vi "Check ABORT.vi"(8 "error in":errorcluster) -> (0 "error out":errorcluster, 3 "ABORT?":bool)   [LabVIEW 2020, in "TALOS.lvlib"]
doc: "Use this VI to check the status of the ABORT SV. It is optimised respect to just opening the SV on the network."
uses:
  TALOS.lvlib
  Classes/Circus Shared Variables/Circus Shared Variables.lvclass/Circus Shared Variables.ctl
  Ancestor/Ancestor/Ancestor.lvclass/Ancestor.ctl
  Generate Error.vi
  FGV/Error Memory/Get Error Description.vi
  Get PC name.vi
  Ancestor/Ancestor/Read ID.vi
  Get Class Name.vi
  <vilib>/Utility/error.llb/Clear Errors.vi
  FGV/Error Memory/Error Memory Core.vi
  <vilib>/AdvancedString/Delimited String to 1D String Array.vi
  Circus Root Path.vi
  FGV/Error Memory/Error Crt Lvl checker.vi
  FGV/Error Memory/Error Memory Core.vi/40c8088d-b597-4017-91af-faa98e00292e.vi
  FGV/Error Memory/Error Memory Core.vi/d4a3ab98-063c-4e44-b43d-fbdcfe6c2be2.vi
  Global Constants.vi
  Global Memory.vi
  <vilib>/Utility/LVClass/Get LV Class Name.vi
  Is in Packed Library.vi
  TALOS Root path.vi
  Read CSV worksheet.vi
  <vilib>/Utility/error.llb/General Error Handler.vi
  Error Log.vi
  Ancestor/Ancestor/Ancestor.lvclass
  <vilib>/Comparison/Equal/Equal Functor/Equal Functor.lvclass
  Classes/Circus Shared Variables/Circus Shared Variables.lvclass
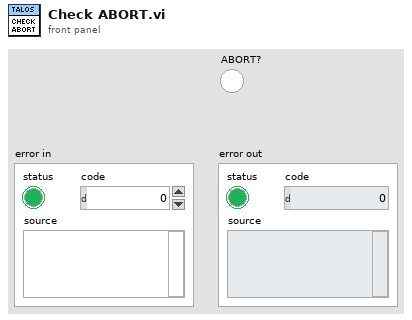
[diagram p1: front panel]
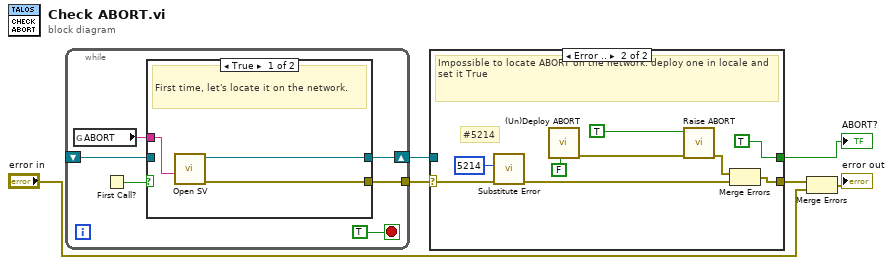
[diagram p0: block diagram]
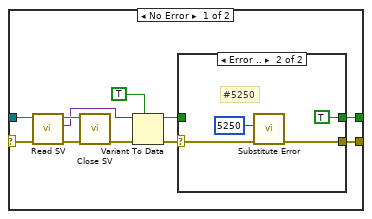
[diagram p2: hidden frame]
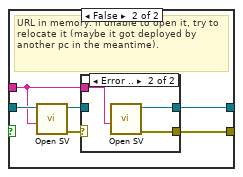
[diagram p4: hidden frame]
diagram:
  n1 = while {
    tunnel: [w12] -> w6
    shift-right: [w11] -> w5
    shift-left: _ -> [w8]
    stop <- TRUE stop-if-true
    n2 = global read "Global Constants.vi" "ABORT"() -> (w7:string)
    n3 = First Call?() -> (First Call?: T/F=w10:bool)
    n4 = case shown="True" w10 {
      tunnel: [w15 w17] -> w12
      tunnel: [w14 w18] -> w11
      tunnel: w8 -> [_ w21]
      tunnel: w7 -> [w13 w16]
      frame True {
        # "First time, let's locate it on the network."
        n5 = call "Open SV.vi"("SV Name"=w13) -> ("error out"=w15:errorcluster, "AEgIS Shared Variables out"=w14:refnum<class "Circus Shared Variables.lvclass">)  [unwired: 9 in]
      }
      frame False {
        # "URL in memory: if unable to open it, try to relocate it (maybe it got deployed by another pc in the meantime)."
        n6 = call "Open SV.vi"("SV Name"=w16, "AEgIS Shared Variables in"=w21) -> ("error out"=w20:errorcluster, "AEgIS Shared Variables out"=w19:refnum<class "Circus Shared Variables.lvclass">)  [unwired: 8 in]
        n7 = case shown="Error .." w20 {
          selector: w20 -> [w22 _]
          tunnel: w19 -> [w23 _]
          tunnel: [w23 w26] -> w18
          tunnel: [w22 w25] -> w17
          tunnel: w16 -> [_ w24]
          frame No Error {
          }
          frame Error {
            n8 = call "Open SV.vi"("SV Name"=w24) -> ("error out"=w25:errorcluster, "AEgIS Shared Variables out"=w26:refnum<class "Circus Shared Variables.lvclass">)  [unwired: 9 in]
          }
        }
      }
    }
  }
  n9 = case shown="Error .." w6 {
    selector: w6 -> [w37 w52]
    tunnel: w5 -> [w34 _]
    tunnel: [w28 TRUE] -> w4
    tunnel: [w27 w45] -> w3
    frame No Error {
      n10 = call "Read SV.vi"("error in (no error)"=w37, "AEgIS Shared Variables in"=w34) -> ("error out"=w36:errorcluster, "Variant"=w32:variant, "AEgIS Shared Variables out"=w35:refnum<class "Circus Shared Variables.lvclass">)  [unwired: 7 in]
      n11 = call "Close SV.vi"("error in (no error)"=w36, "AEgIS Shared Variables in"=w35) -> ("error out"=w33:errorcluster)  [unwired: 7 in, 2 out]
      n12 = Variant To Data(error in=w33, type=TRUE, Variant=w32) -> (data=w29:bool, error out=w30:errorcluster)
      n13 = case shown="Error .." w30 {
        selector: w30 -> [w38 w41]
        tunnel: w29 -> [w39 _]
        tunnel: [w39 TRUE] -> w28
        tunnel: [w38 w40] -> w27
        frame No Error {
        }
        frame Error {
          # "#5250"
          n14 = call "Substitute Error.vi"("error in (no error)"=w41, "Error Code"=5250) -> ("error out"=w40:errorcluster)  [unwired: 9 in]
        }
      }
    }
    frame Error {
      # "#5214"
      # "Impossible to locate ABORT on the network: deploy one in locale and set it True"
      n15 = call "Substitute Error.vi"("error in (no error)"=w52, "Error Code"=5214) -> ("error out"=w50:errorcluster)  [unwired: 9 in]
      n16 = call "(Un)Deploy ABORT.vi"("Undeploy?"=FALSE) -> ("error out"=w48:errorcluster)  [unwired: 10 in]
      n17 = call "Raise ABORT.vi"("error in"=w48, "ABORT?"=TRUE) -> ("error out"=w44:errorcluster)  [unwired: 9 in]
      n18 = Merge Errors(w44, w50) -> (w45:errorcluster)
    }
  }
  "ABORT?" <- w4
  n19 = Merge Errors(w3, "error in") -> (→"error out":errorcluster)
